vi "Move_Arm_to_Camera_Down.vi"(0 "VISA Refnum in":refnum<visa-resource-name>="COM3", 1 "error in":errorcluster) -> (7 "Machine Out":refnum<visa-resource-name>, 8 "error out":errorcluster)   [LabVIEW 2018]
doc: "Example interface for controlling uArm Swift Pro."
panel:
  in  "Stop Program":bool
  in  "Write Buffer":string="G91 G0 X1\n"
  out "read buffer":string
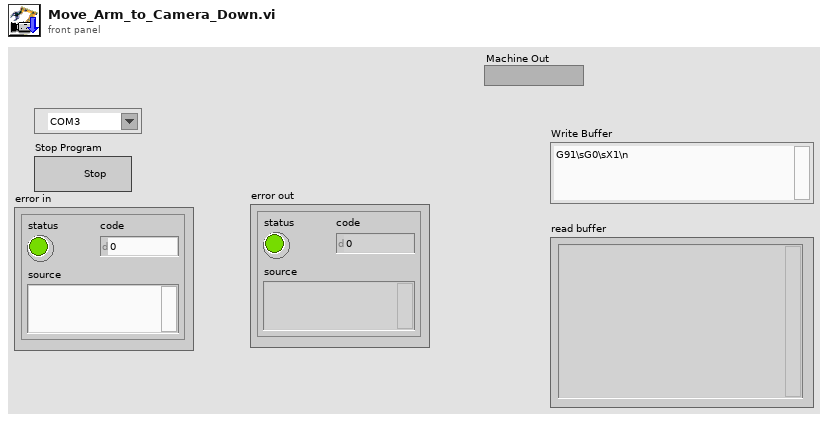
[diagram p1: front panel]
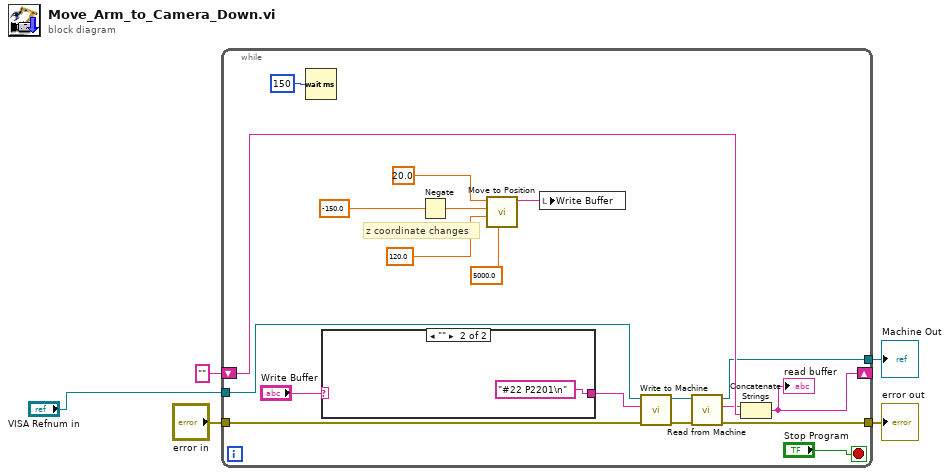
[diagram p0: block diagram]
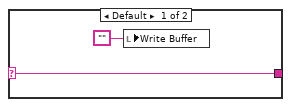
[diagram p2: hidden frame]
diagram:
  n1 = while {
    tunnel: "VISA Refnum in" -> [w20]
    tunnel: "error in" -> [w17]
    shift-right: [w18] -> _
    shift-left: "" -> [w19]
    tunnel: [w16] -> w1
    tunnel: [w12] -> w2
    stop <- "Stop Program" stop-if-true
    # "z coordinate changes"
    n2 = Wait (ms)(milliseconds to wait=u32 150) -> ()  [unwired: 1 out]
    n3 = case shown="\"\"" "Write Buffer" {
      selector: "Write Buffer" -> [w26 _]
      tunnel: [w26 "#22 P2201\n"] -> w22
      frame Default {
        n4 = local write "Write Buffer"("") -> ()
      }
      frame "" {
      }
    }
    n5 = Negate(x=-150.0 ("X-position")) -> (-x=w7:dbl)
    n6 = call "Move to Position.vi"("Speed"=5000.0, "Z-Position"=120.0, "Y-Position"=w7, "X-Position"=20.0 ("Y-position")) -> ("G-Code String"=w9:string)  [unwired: 7 in]
    n7 = local write "Write Buffer"(w9) -> ()
    n8 = call "Write to Machine .vi"("error in (no error)"=w17, "G-Code String In"=w22, "Machine In"=w20) -> ("error out"=w14:errorcluster, "Machine Out"=w13:refnum<visa-resource-name>)  [unwired: 7 in]
    n9 = call "Read from Machine.vi"("error in (no error)"=w14, "Machine In"=w13) -> ("error out"=w12:errorcluster, "read buffer"=w15:string, "Machine Out"=w16:refnum<visa-resource-name>)  [unwired: 7 in]
    n10 = Concatenate Strings(w15, w19) -> (w18:string)
    "read buffer" <- w18
  }
  "error out" <- w2
  "Machine Out" <- w1
